vi "CameraSetupSingleScan.vi"(0 "error in (no error)":errorcluster, 1 "EM adv":bool, 2 "Camera settings":T1={"EM gain?"=FALSE, "EM gain"=100, "preamp gain"=enum."1", "VS speed"=enum."1", "conv HS speed"=enum."1", "EM HS speed"=enum."1"}) -> (3 "error out":errorcluster, 4 "image size":cluster{"xpixels":i32, "ypixels":i32}, 5 "EM gain max":i32, 6 "actual EM gain":i32)   [LabVIEW 2019]
uses:
  <userlib>/atmcd32d.llb/TriggerMode_mode typedef.ctl
  <userlib>/atmcd32d.llb/AcquisitionMode_mode typedef.ctl
  <userlib>/atmcd32d.llb/ReadMode_mode typedef.ctl
  <userlib>/atmcd32d.llb/HSSpeed_type typedef.ctl
  <userlib>/atmcd32d.llb/EMGainMode_mode typedef.ctl
panel:
  out "EM gain min":i32
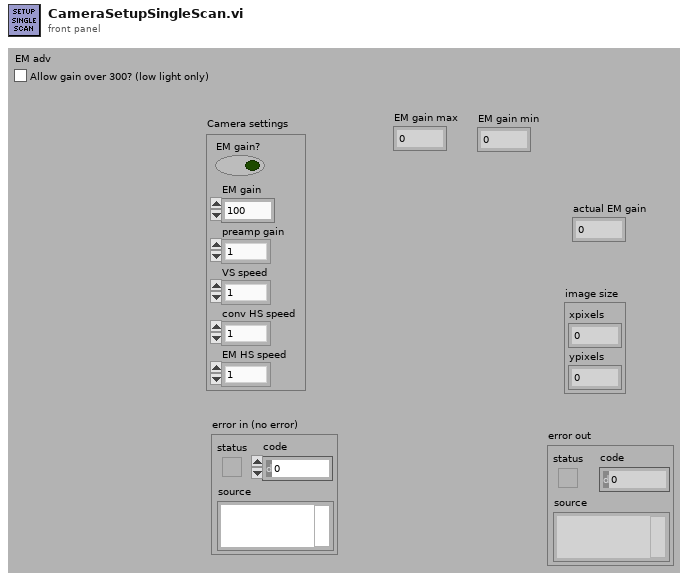
[diagram p1: front panel]
types:
  T1 = cluster{"EM gain?":bool, "EM gain":u16, "preamp gain":enum16{"0", "1", "2", "3"}, "VS speed":enum16{"0", "1", "2", "3"}, "conv HS speed":enum16{"0", "1"}, "EM HS speed":enum16{"0", "1", "2", "3"}}
  T2 = typedef "ReadMode_mode typedef.ctl" = enum16{"Full Vertical Binning", "Multi-Track", "Random-Track", "Single-Track", "Image"}
  T3 = typedef "AcquisitionMode_mode typedef.ctl" = enum16{"Reserved (0)", "Single Scan", "Accumulate", "Kinetics", "Fast Kinetics", "Run Till Abort", "Reserved (6)", "Reserved (7)", "Reserved (8)", "Time Delayed Integration"}
  T4 = typedef "TriggerMode_mode typedef.ctl" = enum16{"Internal", "External", "N/A (2)", "N/A (3)", "N/A (4)", "N/A (5)", "External Start", "External Exposure (Bulb)", "N/A (8)", "External FVB EM", "Software", "N/A (11)", "External Charge Shifting"}
  T5 = typedef "HSSpeed_type typedef.ctl" = enum16{"EM Amp", "Conventional Amp"}
  T6 = typedef "EMGainMode_mode typedef.ctl" = enum16{"8-bit", "12-bit", "Linear", "Real"}
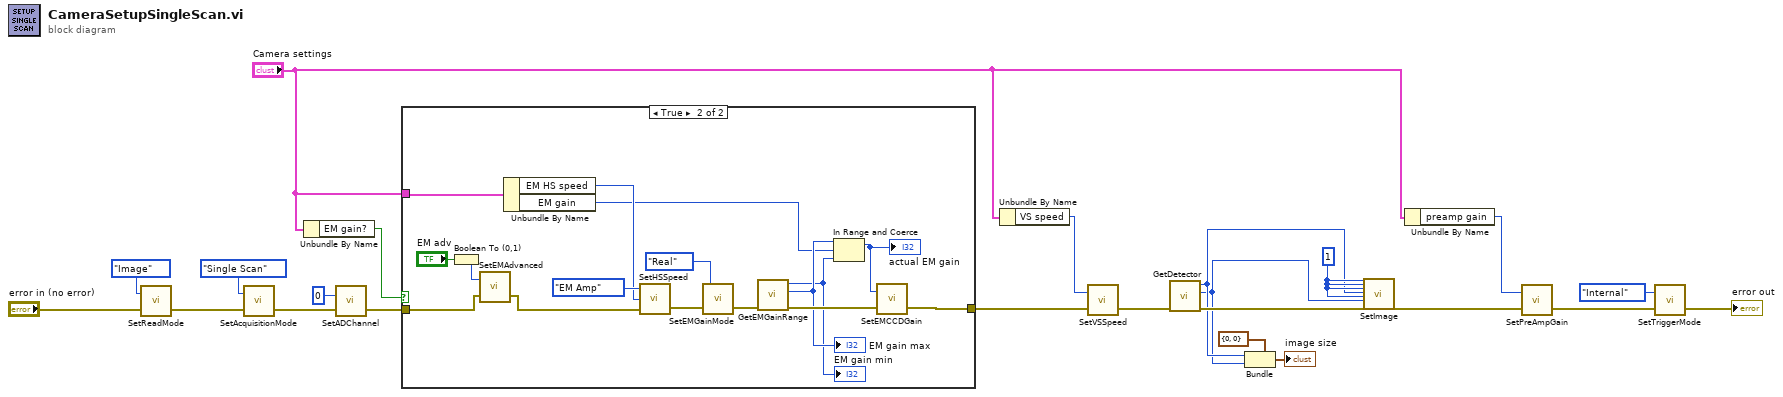
[diagram p0: block diagram]
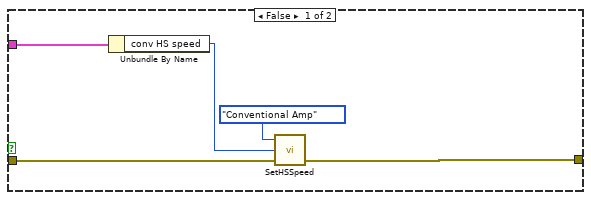
[diagram p2: hidden frame]
diagram:
  w19 = 1
  n1 = call <userlib>:"SetReadMode.vi"("error in (no error)"="error in (no error)", "mode"=ReadMode_mode_typedef."Image") -> ("error out"=w12:errorcluster)  [unwired: 1 out]
  n2 = call <userlib>:"SetAcquisitionMode.vi"("error in (no error)"=w12, "mode"=AcquisitionMode_mode_typedef."Single Scan") -> ("error out"=w13:errorcluster)  [unwired: 1 out]
  n3 = Unbundle By Name("Camera settings") -> ("EM gain?"=w8:bool)
  n4 = call <userlib>:"SetADChannel.vi"("error in (no error)"=w13, "channel"=0) -> ("error out"=w15:errorcluster)  [unwired: 1 out]
  n5 = case shown="True" w8 {
    tunnel: w15 -> [w27 w32]
    tunnel: [w26 w36] -> w16
    tunnel: "Camera settings" -> [w25 w35]
    frame False {
      n6 = Unbundle By Name(w25) -> ("conv HS speed"=w24:enum16{"0", "1"})
      n7 = call <userlib>:"SetHSSpeed.vi"("error in (no error)"=w27, "index"=w24, "type"=HSSpeed_type_typedef."Conventional Amp") -> ("error out"=w26:errorcluster)  [unwired: 1 in, 1 out]
    }
    frame True {
      n8 = Boolean To (0,1)(Boolean="EM adv") -> (0, 1=w29:i16)
      n9 = call <userlib>:"SetEMAdvanced.vi"("error in (no error)"=w32, "state"=w29) -> ("error out"=w31:errorcluster)  [unwired: 1 out]
      n10 = Unbundle By Name(w35) -> ("EM HS speed"=w34:enum16{"0", "1", "2", "3"}, "EM gain"=w33:u16)
      n11 = call <userlib>:"SetHSSpeed.vi"("error in (no error)"=w31, "index"=w34, "type"=HSSpeed_type_typedef."EM Amp") -> ("error out"=w44:errorcluster)  [unwired: 1 in, 1 out]
      n12 = call <userlib>:"SetEMGainMode.vi"("error in (no error)"=w44, "mode"=EMGainMode_mode_typedef."Real") -> ("error out"=w41:errorcluster)  [unwired: 1 out]
      n13 = call <userlib>:"GetEMGainRange.vi"("error in (no error)"=w41) -> ("error out"=w40:errorcluster, "high"=w39:i32, "low"=w38:i32)  [unwired: 3 in, 1 out]
      "EM gain max" <- w39
      "EM gain min" <- w38
      n14 = In Range and Coerce(upper limit=w39, x=w33, lower limit=w38) -> (coerced(x)=w37:i32)  [unwired: 1 out]
      "actual EM gain" <- w37
      n15 = call <userlib>:"SetEMCCDGain.vi"("error in (no error)"=w40, "gain"=w37) -> ("error out"=w36:errorcluster)  [unwired: 1 out]
    }
  }
  n16 = Unbundle By Name("Camera settings") -> ("VS speed"=w7:enum16{"0", "1", "2", "3"})
  n17 = call <userlib>:"SetVSSpeed.vi"("error in (no error)"=w16, "index"=w7) -> ("error out"=w18:errorcluster)  [unwired: 1 out]
  n18 = call <userlib>:"GetDetector.vi"("error in (no error)"=w18) -> ("error out"=w17:errorcluster, "ypixels"=w3:i32, "xpixels"=w4:i32)  [unwired: 3 in, 1 out]
  n19 = Bundle(cluster=cluster{"xpixels":i32, "ypixels":i32} {"xpixels"=0, "ypixels"=0} ("image size"), "xpixels"=w4, "ypixels"=w3) -> (→"image size":cluster{"xpixels":i32, "ypixels":i32})
  n20 = call <userlib>:"SetImage.vi"("hbin"=w19, "vbin"=w19, "hstart"=w19, "hend"=w4, "vstart"=w19, "vend"=w3, "error in (no error)"=w17) -> ("error out"=w20:errorcluster)  [unwired: 19 in, 1 out]
  n21 = Unbundle By Name("Camera settings") -> ("preamp gain"=w6:enum16{"0", "1", "2", "3"})
  n22 = call <userlib>:"SetPreAmpGain.vi"("error in (no error)"=w20, "index"=w6) -> ("error out"=w22:errorcluster)  [unwired: 1 out]
  n23 = call <userlib>:"SetTriggerMode.vi"("error in (no error)"=w22, "mode"=TriggerMode_mode_typedef."Internal") -> ("error out"=→"error out":errorcluster)  [unwired: 1 out]
